vi "SIM Compute Ft.vi"(4 "reset?":bool, 6 "F_current":dbl[](array[numeric]) format="%.16e", 7 "t_current":dbl) -> (0 "Ft":dbl[](array[numeric]), 1 "done?":bool, 2 "F0":dbl[](array[numeric]), 3 "t_next":dbl)   [LabVIEW 2017]
uses:
  <vilib>/Simulation/ContinuousLinear/Implementation/Shared/Solvers/SIM BDF.llb/SIM BDF jacobian stages.ctl
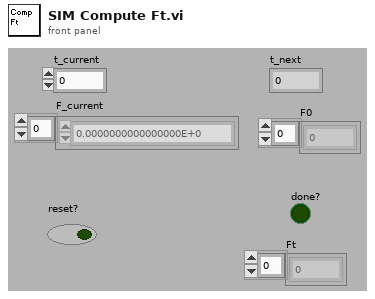
[diagram p1: front panel]
types:
  T1 = typedef "SIM BDF jacobian stages.ctl" = enum16{"first output", "second output"}
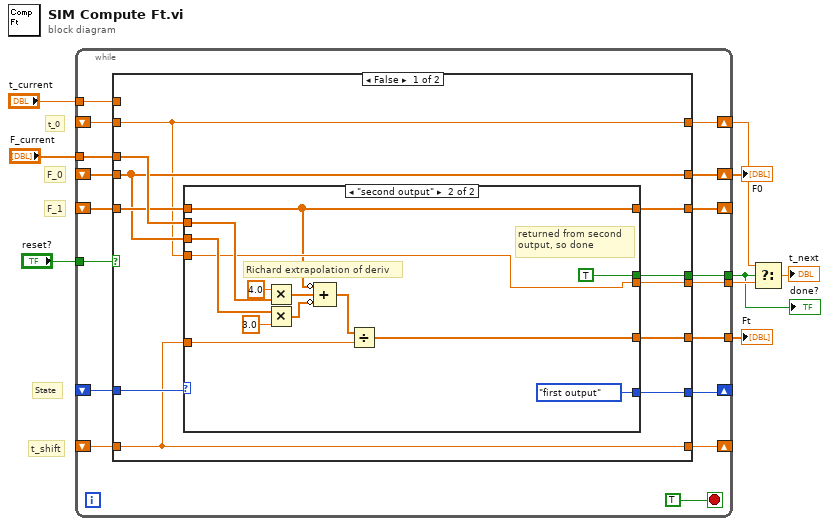
[diagram p0: block diagram]
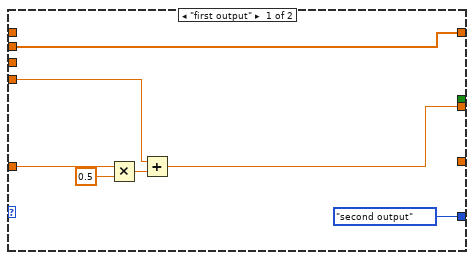
[diagram p2: hidden frame]
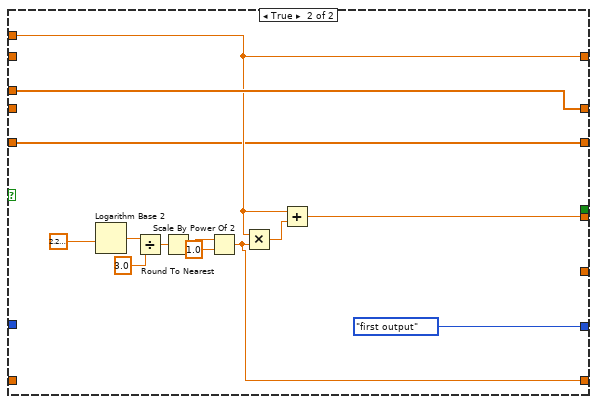
[diagram p3: hidden frame]
diagram:
  # "t_0"
  # "F_1"
  # "F_0"
  # "State"
  # "t_shift"
  n1 = while {
    tunnel: "t_current" -> [w25]
    tunnel: "reset?" -> [w26]
    tunnel: [w24] -> w6
    shift-right: [w23] -> _
    shift-left: _ -> [w11]
    shift-right: [w22] -> _
    shift-left: _ -> [w17]
    shift-right: [w21] -> w1
    shift-left: _ -> [w14]
    shift-right: [w12] -> _
    shift-left: _ -> [w13]
    tunnel: "F_current" -> [w20]
    shift-right: [w19] -> w5
    shift-left: _ -> [w18]
    tunnel: [w15] -> w2
    tunnel: [w10] -> w3
    stop <- TRUE stop-if-true
    n2 = case shown="False" w26 {
      tunnel: w25 -> [_ w60]
      tunnel: [w29 w64] -> w24
      tunnel: [w28 w63] -> w23
      tunnel: [w36 SIM_BDF_jacobian_stages."first output" ("Jacobian computation stage")] -> w22
      tunnel: [w32 w61] -> w21
      tunnel: w20 -> [w34 w61]
      tunnel: [w30 w60] -> w19
      tunnel: w18 -> [w30 _]
      tunnel: w17 -> [w37 _]
      tunnel: [w35 _] -> w15
      tunnel: w14 -> [w32 _]
      tunnel: w13 -> [w33 w59]
      tunnel: [w31 w59] -> w12
      tunnel: w11 -> [w28 _]
      tunnel: [w27 _] -> w10
      frame False {
        n3 = case shown="\"second output\"" w37 {
          tunnel: [SIM_BDF_jacobian_stages."second output" ("Jacobian computation stage") SIM_BDF_jacobian_stages."first output" ("Jacobian computation stage")] -> w36
          tunnel: [_ TRUE] -> w35
          tunnel: w34 -> [w43 w51]
          tunnel: w33 -> [_ w45]
          tunnel: w32 -> [_ w49]
          tunnel: [w43 w45] -> w31
          tunnel: w30 -> [w39 w46]
          tunnel: w28 -> [w42 w48]
          tunnel: [w38 w46] -> w29
          tunnel: [_ w47] -> w27
          frame "first output" {
            n4 = Multiply(x=w42, y=0.5) -> (x*y=w40:dbl)
            n5 = Add(x=w39, y=w40) -> (x+y=w38:dbl)
          }
          frame "second output" {
            # "Richard extrapolation of deriv"
            # "returned from second\noutput, so done"
            n6 = Multiply(x=4.0, y=w51) -> (x*y=w52:dbl[])
            n7 = Multiply(x=w49, y=3.0) -> (x*y=w53:dbl[])
            n8 = Compound Arithmetic op=ADD(invert w45, w52, invert w53) -> (w54:dbl[])
            n9 = Divide(x=w54, y=w48) -> (x/y=w47:dbl[])
          }
        }
      }
      frame True {
        n10 = Logarithm Base 2(1:2.220446049250313e-16) -> (0:w70:dbl)
        n11 = Divide(x=w70, y=3.0) -> (x/y=w68:dbl)
        n12 = Round To Nearest(number=w68) -> (nearest integer value=w67:dbl)
        n13 = Scale By Power Of 2(n=w67, x=1.0) -> (x*2^n=w63:dbl)
        n14 = Multiply(x=w60, y=w63) -> (x*y=w65:dbl)
        n15 = Add(x=w60, y=w65) -> (x+y=w64:dbl)
      }
    }
  }
  "Ft" <- w3
  "done?" <- w2
  "F0" <- w1
  n16 = Select(t=w5, s=w2, f=w6) -> (s? t:f=→"t_next":dbl)
